vi "GDSLvClass_ReadClassType.vi"(0 "Class Refnum In":refnum<vi>, 5 "error in (no error)":errorcluster) -> (14 "Class Refnum Out":refnum<vi>, 15 "ClassSettings":T1, 19 "error out":errorcluster)   [LabVIEW 2020]
uses:
  <resource>/Framework/Providers/Open_GDS/ClassProviders/Common/LvClass_class/GDSLvCLass_ClassSettingsType.ctl
  <resource>/Framework/Providers/Open_GDS/ClassProviders/Common/LvClass_class/GDSLvClass_PlugIn.ctl
  <resource>/Framework/Providers/Open_GDS/ClassProviders/Common/LvClass_class/GDSLvClass_PlugInTypes.ctl
  <resource>/Framework/Providers/Open_GDS/ClassProviders/Common/LvClass_class/GDSLvClass_ClassTypeSettingNames.ctl
  <resource>/Framework/Providers/Open_GDS/ClassProviders/Provider_LvNativeClass/LvNativeProviderName.ctl
  <resource>/Framework/Providers/Open_GDS/ClassProviders/Common/ScriptingFunctions/Scripting_ConnectorPanePatternType.ctl
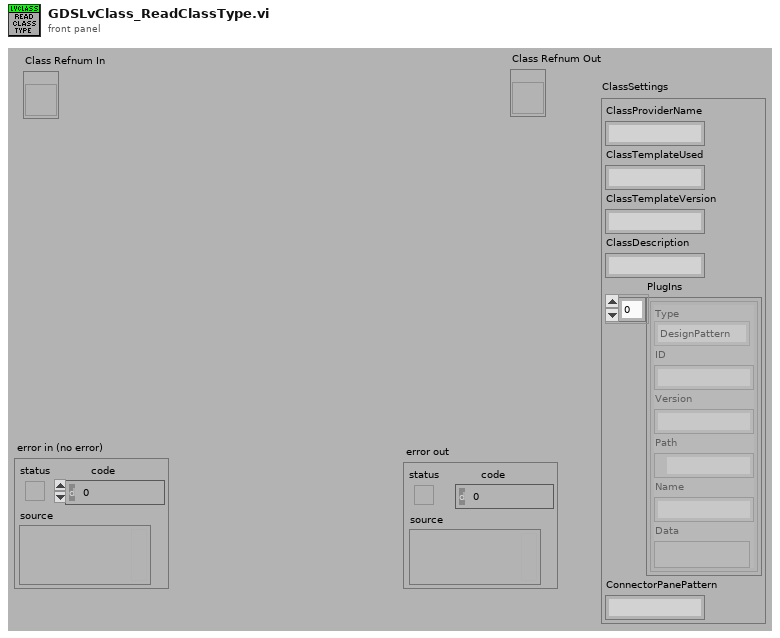
[diagram p1: front panel]
types:
  T1 = typedef "GDSLvCLass_ClassSettingsType.ctl" = cluster{"ClassProviderName":string, "ClassTemplateUsed":string, "ClassTemplateVersion":string, "ClassDescription":string, "PlugIns":T2[], "ConnectorPanePattern":string}
  T2 = typedef "GDSLvClass_PlugIn.ctl" = cluster{"Type":T3, "ID":string, "Version":string, "Path":path, "Name":string, "Data":variant}
  T3 = typedef "GDSLvClass_PlugInTypes.ctl" = enum16{"DesignPattern", "MethodTypes"}
  T4 = typedef "LvNativeProviderName.ctl" = enum16{"Endevo LabVIEW Native"}
  T5 = typedef "GDSLvClass_ClassTypeSettingNames.ctl" = enum16{"EndevoGOOP_ClassProvider", "EndevoGOOP_TemplateUsed", "EndevoGOOP_TemplateVersion", "EndevoGOOP_PlugIns", "EndevoGOOP_ConnectorPanePattern"}
  T6 = typedef "Scripting_ConnectorPanePatternType.ctl" = u16
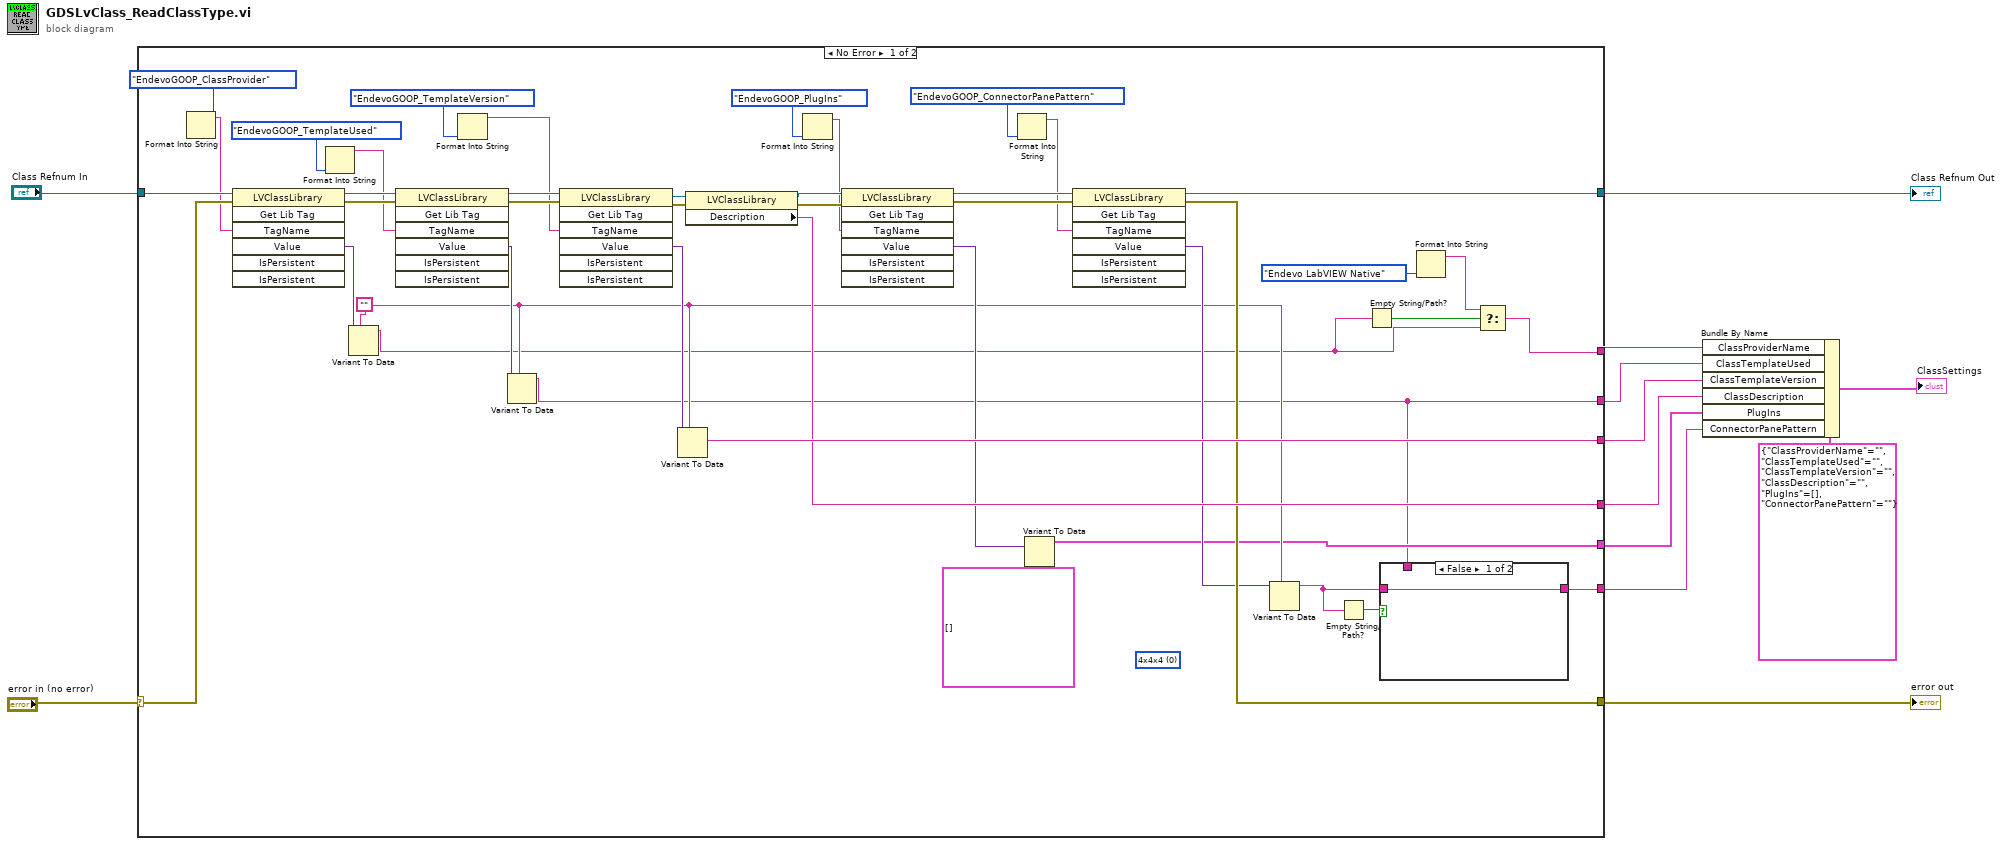
[diagram p0: block diagram]
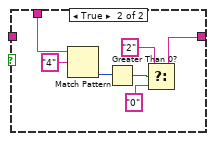
[diagram p2: hidden frame]
diagram:
  n1 = case shown="No Error" "error in (no error)" {
    selector: "error in (no error)" -> [w55 w65]
    tunnel: [w29 w65] -> w11
    tunnel: "Class Refnum In" -> [w50 w64]
    tunnel: [w28 w64] -> w9
    tunnel: [w15 _] -> w7
    tunnel: [w47 _] -> w6
    tunnel: [w18 _] -> w1
    tunnel: [w44 _] -> w5
    tunnel: [w23 _] -> w3
    tunnel: [w19 _] -> w2
    frame No Error {
      (unwired) T6 0 items=["4x4x4", "5x6x5", "6x8x6"] ("Pattern")
      w24 = ""
      n2 = Format Into String(GDSLvClass_ClassTypeSettingNames."EndevoGOOP_ClassProvider" ("ClassTypeSettingNames")) -> (resulting string=w39:string)  [unwired: 3 in, 1 out]
      n3 = invoke class="LVClassLibrary" method="Get Lib Tag"(reference=w50, error in=w55, "TagName"=w39) -> (reference out=w54:refnum<vi>, error out=w53:errorcluster, "Value"=w52:variant)  [unwired: 4 in, 4 out]
      n4 = Format Into String(GDSLvClass_ClassTypeSettingNames."EndevoGOOP_TemplateUsed" ("ClassTypeSettingNames")) -> (resulting string=w37:string)  [unwired: 3 in, 1 out]
      n5 = Variant To Data(type=w24, Variant=w52) -> (data=w16:string)  [unwired: 1 in, 1 out]
      n6 = invoke class="LVClassLibrary" method="Get Lib Tag"(reference=w54, error in=w53, "TagName"=w37) -> (reference out=w49:refnum<vi>, error out=w48:errorcluster, "Value"=w51:variant)  [unwired: 4 in, 4 out]
      n7 = Format Into String(GDSLvClass_ClassTypeSettingNames."EndevoGOOP_TemplateVersion" ("ClassTypeSettingNames")) -> (resulting string=w38:string)  [unwired: 3 in, 1 out]
      n8 = Variant To Data(type=w24, Variant=w51) -> (data=w18:string)  [unwired: 1 in, 1 out]
      n9 = invoke class="LVClassLibrary" method="Get Lib Tag"(reference=w49, error in=w48, "TagName"=w38) -> (reference out=w46:refnum<vi>, error out=w45:errorcluster, "Value"=w43:variant)  [unwired: 4 in, 4 out]
      n10 = Variant To Data(type=w24, Variant=w43) -> (data=w47:string)  [unwired: 1 in, 1 out]
      n11 = property class="LVClassLibrary"(reference=w46, error in=w45) -> (reference out=w36:refnum<vi>, error out=w35:errorcluster, "Description"=w44:string)
      n12 = Format Into String(GDSLvClass_ClassTypeSettingNames."EndevoGOOP_PlugIns" ("ClassTypeSettingNames")) -> (resulting string=w33:string)  [unwired: 3 in, 1 out]
      n13 = invoke class="LVClassLibrary" method="Get Lib Tag"(reference=w36, error in=w35, "TagName"=w33) -> (reference out=w31:refnum<vi>, error out=w30:errorcluster, "Value"=w32:variant)  [unwired: 4 in, 4 out]
      n14 = Format Into String(GDSLvClass_ClassTypeSettingNames."EndevoGOOP_ConnectorPanePattern" ("ClassTypeSettingNames")) -> (resulting string=w26:string)  [unwired: 3 in, 1 out]
      n15 = Variant To Data(type=T2[] [] ("PlugIns"), Variant=w32) -> (data=w23:T2[])  [unwired: 1 in, 1 out]
      n16 = invoke class="LVClassLibrary" method="Get Lib Tag"(reference=w31, error in=w30, "TagName"=w26) -> (reference out=w28:refnum<vi>, error out=w29:errorcluster, "Value"=w25:variant)  [unwired: 4 in, 4 out]
      n17 = Variant To Data(type=w24, Variant=w25) -> (data=w20:string)  [unwired: 1 in, 1 out]
      n18 = Empty String/Path?(string/path=w20) -> (empty?=w21:bool)
      n19 = Empty String/Path?(string/path=w16) -> (empty?=w17:bool)
      n20 = case shown="False" w21 {
        tunnel: w20 -> [w56 _]
        tunnel: [w56 w59] -> w19
        tunnel: w18 -> [_ w63]
        frame False {
        }
        frame True {
          n21 = Match Pattern(string=w63, regular expression="4") -> (offset past match=w61:i32)  [unwired: 1 in, 3 out]
          n22 = Greater Than 0?(x=w61) -> (x > 0?=w60:bool)
          n23 = Select(t="2", s=w60, f="0" ("regular expression")) -> (s? t:f=w59:string)
        }
      }
      n24 = Format Into String(LvNativeProviderName."Endevo LabVIEW Native" ("ProviderName")) -> (resulting string=w13:string)  [unwired: 3 in, 1 out]
      n25 = Select(t=w13, s=w17, f=w16) -> (s? t:f=w15:string)
    }
    frame Error {
    }
  }
  "Class Refnum Out" <- w9
  "error out" <- w11
  n26 = Bundle By Name(cluster=T1 {"ClassProviderName"="", "ClassTemplateUsed"="", "ClassTemplateVersion"="", "ClassDescription"="", "PlugIns"=[], "ConnectorPanePattern"=""} ("ClassSettings"), "ClassProviderName"=w7, "ClassTemplateUsed"=w1, "ClassTemplateVersion"=w6, "ClassDescription"=w5, "PlugIns"=w3, "ConnectorPanePattern"=w2) -> (→"ClassSettings":T1)
